vi "Display ViewableActor.vi"(8 "error in (no error)":errorcluster, 10 "ViewableActor":refnum<class "Message Enqueuer.lvclass">, 11 "SubPanel Grid View in":refnum<class "SubPanel Grid View.lvclass">) -> (0 "error out":errorcluster, 3 "SubPanel Grid View out":refnum<class "SubPanel Grid View.lvclass">)   [LabVIEW 2012, in "Win8uiDemo.lvlib" / "SubPanel Grid View.lvclass"]
uses:
  SubPanel Grid View.lvclass
  <vilib>/ActorFramework/Message Enqueuer/Message Enqueuer.lvclass
  SubPanel Grid View.lvclass/SubPanel Grid View.ctl
  Win8uiFramework/Insert Into SubPanel Msg.lvclass/Insert Into SubPanel Msg.ctl
  <vilib>/ActorFramework/Message Enqueuer/Message Enqueuer.lvclass/Message Enqueuer.ctl
  Read ViewableActor Enqueuers.vi
  SubPanel 3x3 View/Read SubPanel Array.vi
  Read NextIndex.vi
  Write ViewableActor Enqueuers.vi
  Write NextIndex.vi
  <vilib>/ActorFramework/Message Enqueuer/Enqueue.vi
  <vilib>/ActorFramework/Message Priority Queue/Priority Enqueue.vi
  Win8uiFramework/Insert Into SubPanel Msg.lvclass
  <vilib>/ActorFramework/Stop Msg/Stop Msg.lvclass
  Win8uiFramework/Win8uiFramework.lvlib
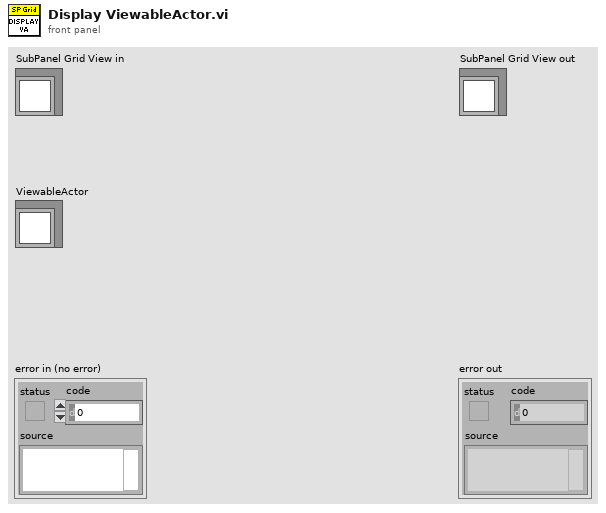
[diagram p1: front panel]
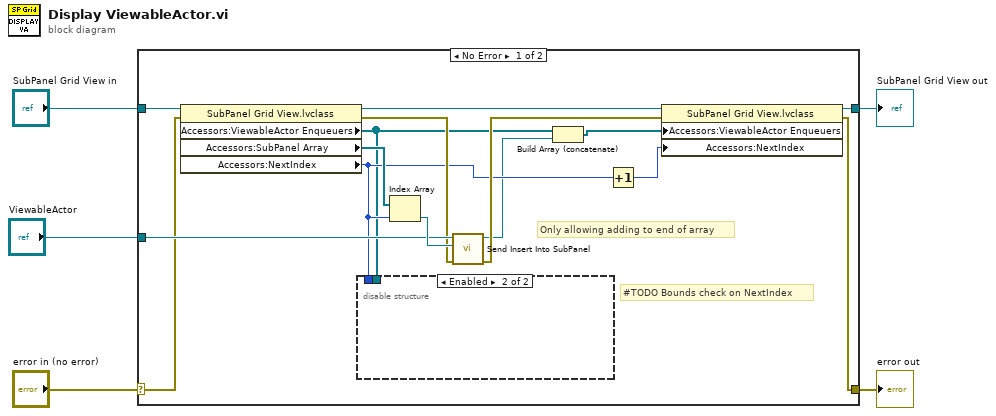
[diagram p0: block diagram]
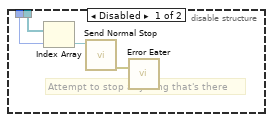
[diagram p2: hidden frame]
diagram:
  n1 = case shown="No Error" "error in (no error)" {
    selector: "error in (no error)" -> [w14 w26]
    tunnel: [w11 w26] -> w4
    tunnel: [w15 w25] -> w2
    tunnel: "SubPanel Grid View in" -> [w20 w25]
    tunnel: "ViewableActor" -> [w16 _]
    frame No Error {
      # "Only allowing adding to end of array"
      # "#TODO Bounds check on NextIndex"
      n2 = property class="SubPanel Grid View.lvclass"(reference=w20, error in=w14) -> (reference out=w19:refnum<class "SubPanel Grid View.lvclass">, error out=w13:errorcluster, "Accessors:ViewableActor Enqueuers"=w8:refnum<class "Message Enqueuer.lvclass">[], "Accessors:SubPanel Array"=w18:refnum<vi>[], "Accessors:NextIndex"=w9:i32)
      n3 = disable-structure shown="Enabled" {
        disable-tunnel: w8 -> [w24 _]
        disable-tunnel: w9 -> [w21 _]
        frame Disabled {
          # "Attempt to stop anything that's there"
          n4 = Index Array(array=w24, index=w21) -> (element=w23:refnum<class "Message Enqueuer.lvclass">)
          n5 = call <vilib>:"Send Normal Stop.vi"("Message Enqueuer"=w23) -> ("error out"=w22:errorcluster)  [unwired: 10 in]
          n6 = call "Error Eater.vi"("error in (no error)"=w22) -> ()  [unwired: 2 in]
        }
        frame Enabled {
        }
      }
      n7 = Index Array(array=w18, index=w9) -> (element=w17:refnum<vi>)
      n8 = call "Send Insert Into SubPanel.vi"("error in (no error)"=w13, "SubPanel Ref"=w17, "Message Enqueuer"=w16) -> ("error out"=w12:errorcluster, "Message Enqueuer out"=w7:refnum<class "Message Enqueuer.lvclass">)  [unwired: 7 in]
      n9 = Build Array (concatenate)(w8, w7) -> (w6:refnum<class "Message Enqueuer.lvclass">[])
      n10 = Increment(x=w9) -> (x+1=w10:i32)
      n11 = property class="SubPanel Grid View.lvclass"(reference=w19, error in=w12, "Accessors:ViewableActor Enqueuers"=w6, "Accessors:NextIndex"=w10) -> (reference out=w15:refnum<class "SubPanel Grid View.lvclass">, error out=w11:errorcluster)
    }
    frame Error {
    }
  }
  "error out" <- w4
  "SubPanel Grid View out" <- w2
